vi "Write Reset Counter Enable.vi"(8 "error in":errorcluster, 11 "MB_TCP session in":refnum<class "MB_Master_TCP.lvclass">) -> (0 "error out":errorcluster, 3 "MB session out":refnum<class "MB_Master_TCP.lvclass">)   [LabVIEW 2024, in "Bronkhorst Flexi-Flow ModbusTCP API.lvlib"]
uses:
  Bronkhorst Flexi-Flow ModbusTCP API.lvlib
  <vilib>/Plasmionique/MB Master/MB_Master_TCP/MB_Master_TCP.lvclass
  PDU Address Char 8-bit Params--ring.ctl
  Write Char Register.vi
  Read Char Register.vi
panel:
  in  "Unsigned Char":string
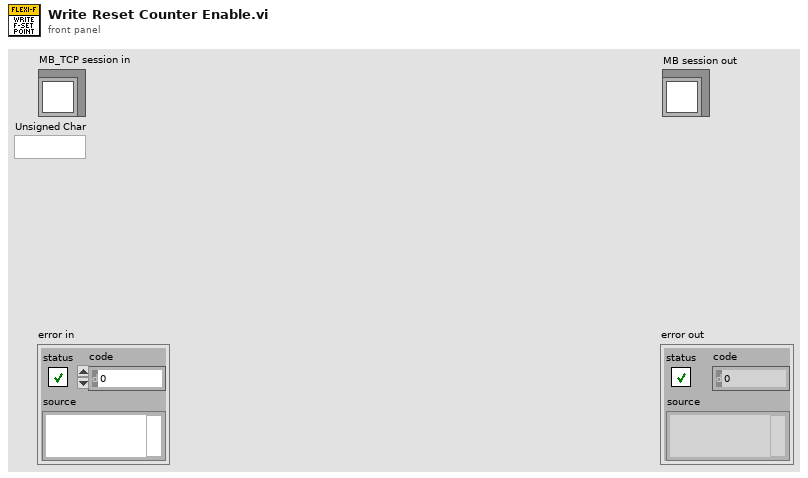
[diagram p1: front panel]
types:
  T1 = typedef "Bronkhorst Flexi-Flow ModbusTCP API.lvlib/PDU Address Char 8-bit Params--ring.ctl" = u16
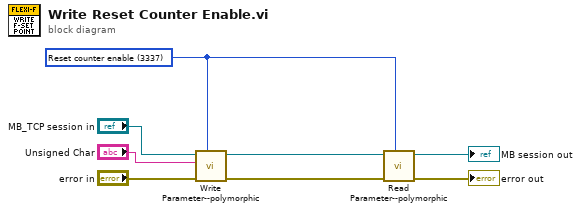
[diagram p0: block diagram]
diagram:
  w1 = T1 3337 items=["Wink"=0, "Control mode"=36, "Alarm mode"=3107, "Alarm setpoint"=3109, "Reset alarm enable"=3113, "Counter unit index"=3330, "Counter setpoint mode"=3333, "Counter mode"=3336, "Reset counter enable"=3337, "Modbus slave address"=4010] ("PDU Address Char 8-bit")
  n1 = call-poly "Write Parameter--polymorphic.vi"("PDU Address Char 8-bit"=w1, "error in"="error in", "Unsigned Char"="Unsigned Char", "MB_TCP session in"="MB_TCP session in") -> ("error out"=w4:errorcluster, "MB session out"=w6:refnum<class "MB_Master_TCP.lvclass">)  [unwired: 6 in]
  n2 = call-poly "Read Parameter--polymorphic.vi"("PDU Address Char 8-bit"=w1, "error in"=w4, "MB_TCP session in"=w6) -> ("error out"=→"error out":errorcluster, "MB session out"=→"MB session out":refnum<class "MB_Master_TCP.lvclass">)  [unwired: 6 in, 1 out]
